vi "ziExample-Module-MDS_DAQ.vi"() -> ()   [LabVIEW 2009]
doc: "This examples allows to control a Zurich Instruments device via a LabOne Labview API. \nThis vi enables the multi-device synchronisation of two ZI instruments of the same family.\n\n© Zurich Instruments AG, www.zhinst.com"
uses:
  <instrlib>/Zurich Instruments LabOne/Public/Modules/ziTypeModEnum.ctl
  <instrlib>/Zurich Instruments LabOne/Public/Modules/ziModSetValueDouble.vi
  <instrlib>/Zurich Instruments LabOne/Public/Modules/ziModSetValueDoubleArray.vi
  <instrlib>/Zurich Instruments LabOne/Public/Modules/ziModSetValueBinary.vi
  <instrlib>/Zurich Instruments LabOne/Public/Modules/ziModGetDoubleData.vi
  <instrlib>/Zurich Instruments LabOne/Public/Utility/ziTicksToS_vector.vi
  <instrlib>/Zurich Instruments LabOne/Zurich Instruments LabOne.lvlib
panel:
  in  "subscribe":string[](array[string])=["demods/0/sample.R", "demods/0/sample.AuxIn1"] caption="Subscribe Paths"
  out "DoubleSample":T1
  in  "stop":bool
  out "XY Graph":cluster{"Timestamp(s)":dbl[], "Value":dbl[]}[](graph)
  in  "noofpoints":i32=10 caption="Number of Points"
  in  "duration":dbl=1.0 caption="Duration (s)"
  out "Error Out":errorcluster
  in  "Slaves":string[](array[string])=["dev"]
  out "Status":dbl
  out "Message":string
  in  "Master":string="dev"
  # "ziExample-Module-MDS_DAQ.vi\nRequirements: 2x(MFLI or UHF or HDAWG )\nsee block diagram for VI description"
  # "Tested Devices:\n\n- MFLI\n- UHF"
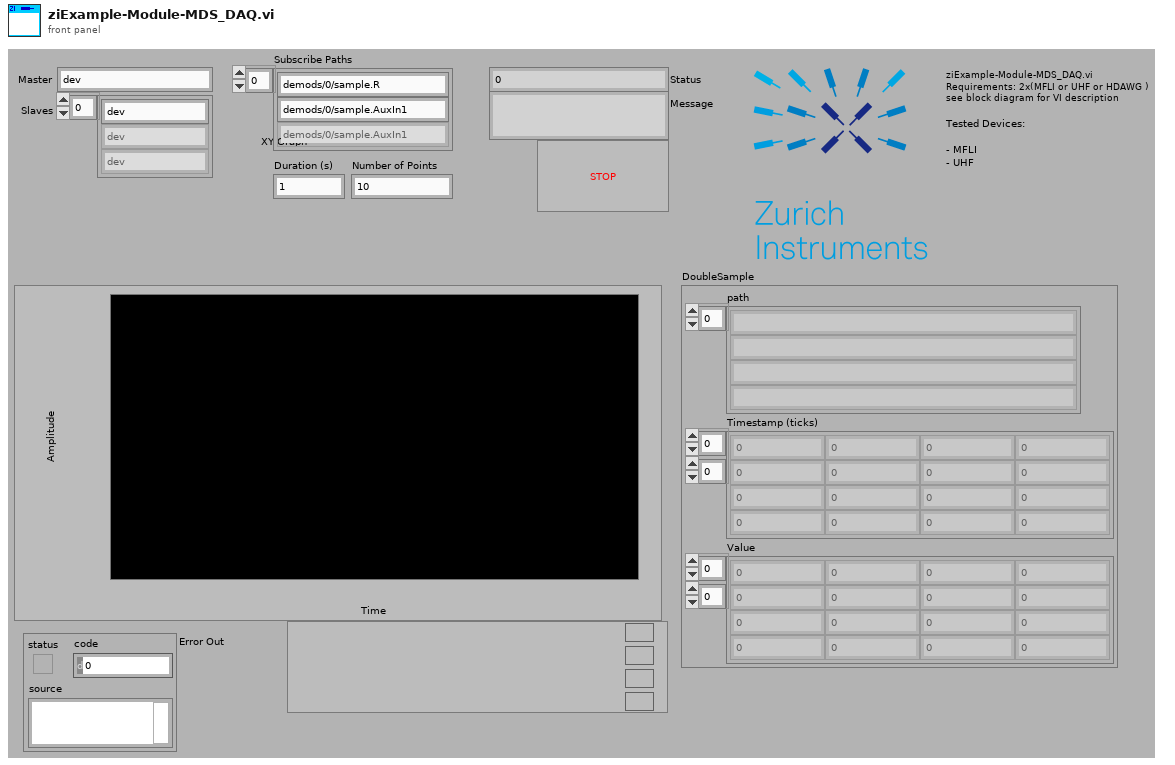
[diagram p1: front panel]
types:
  T1 = cluster{"path":string[], "Timestamp (ticks)":u64[][], "Value":dbl[][]}
  T2 = typedef "Zurich Instruments LabOne.lvlib/ziTypeModEnum.ctl" = u16
  T3 = typedef "Zurich Instruments LabOne.lvlib/ziTypeHandle.ctl" = cluster{"handleValid":bool, "Conn":u64, "Path Prefix":string, "Handle":u64, "Connected":bool, "Clockbase(s)":dbl}
  T4 = typedef "Zurich Instruments LabOne.lvlib/ziTypeModHandle.ctl" = cluster{"handleValid":bool, "Conn":u64, "ModHandle":u64, "moduleID":string, "Path Prefix":string}
  T5 = typedef "Zurich Instruments LabOne.lvlib/ziTypeModResults.ctl" = cluster{"PathArray":string[], "ValueType":T6, "NoOfResults":u64, "ziGenericHeader":T7[]}
  T6 = typedef "Zurich Instruments LabOne.lvlib/ziTypePollType.ctl" = enum16{"NONE", "DOUBLE_DATA", "INTEGER_DATA", "DEMOD_SAMPLE", "SCOPE_WAVE_HF2", "AUXIN_SAMPLE", "DIO_SAMPLE", "BYTE_ARRAY", "PWA_WAVE", "9", "10", "11", "12", "13", "14", "15", "TREE_CHANGE_DEPRI", "17", "ERROR", "19", "20", "21", "22", "23", "24", "25", "26", "27", "28", "29", "30", "31", "DOUBLE_DATA_TS", "INTEGER_DATA_TS", "34", "SCOPE_WAVE", "SCOPE_WAVE_EX", "37", "BYTE_ARRAY_TS", "39", "40", "41", "42", "43", "44", "45", "CNT_DATA", "47", "TREE_CHANGE", "49", "50", "51", "52", "53", "54", "55", "56", "57", "58", "59", "60", "61", "62", "63", "SWEEPER_DATA", "SPECTRUM_DATA", "ADVISOR_DATA", "VECTOR_DATA", "IMP_DATA"}
  T7 = typedef "Zurich Instruments LabOne.lvlib/ziTypeModGenericHeader.ctl" = cluster{"HeaderType":enum8{"HEADER_TYPE_NONE", "HEADER_TYPE_SWTRIGGER", "HEADER_TYPE_SWEEPER"}, "SampleFormat":u8, "SystemTime":timestamp, "CreatedTimeStamp":u64, "ChangedTimeStamp":u64, "Flags":u32, "ChunkSizeBytes":u64, "Name":string, "Status":u32, "GroupIndex":u32, "Color":u32, "ActiveRow":u32, "TriggerNumber":u64, "GridRows":u32, "GridCols":u32, "GridMode":u32, "GridOperation":u32, "GridDirection":u32, "GridRepetitions":u32, "GridColDelta":dbl, "GridColOffset":dbl, "GridRowDelta":dbl, "GridRowOffset":dbl, "Bandwidth":dbl, "Center":dbl, "Nenbw":dbl}
  T8 = typedef "Zurich Instruments LabOne.lvlib/ziTypeDoubleDataTS.ctl" = cluster{"Timestamp (ticks)":u64[], "Value":dbl[]}
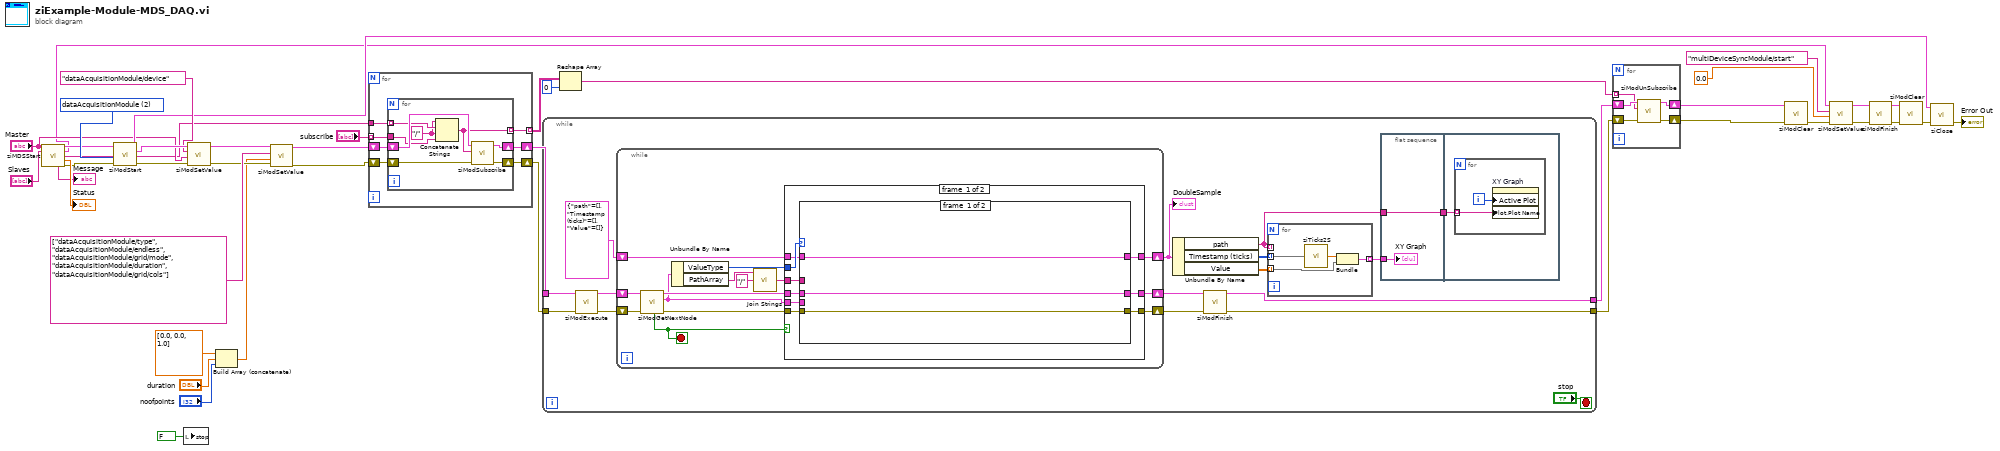
[diagram p0: block diagram]
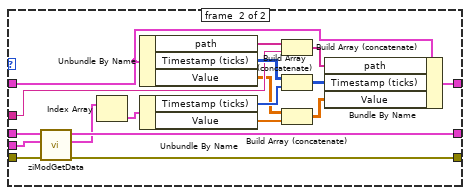
[diagram p2: hidden frame]
diagram:
  w20 = T2 2 items=["sweep", "scopeModule", "dataAcquisitionModule", "pidAdvisor", "awgModule", "impedanceModule", "multiDeviceSyncModule", "zoomFFT", "trigger", "deviceSettings", "record"] ("module Id")
  n1 = call <instrlib>:"ziMDSStart.vi"("Master"="Master", "Slaves"="Slaves") -> ("Handle Out"=w14:T3, "ModHandle Out"=w6:T4, "MDS_Devices"=w10:string[], "Status"=→"Status":dbl, "Message"=→"Message":string, "Error Out"=w13:errorcluster)  [unwired: 8 in]
  n2 = call <instrlib>:"ziModStart.vi"("Error In"=w13, "module Id"=w20, "Handle In"=w14) -> ("Error Out"=w34:errorcluster, "ModHandle Out"=w35:T4, "Handle Out"=w16:T3)  [unwired: 6 in]
  n3 = local write "stop"(FALSE ("run")) -> ()
  n4 = call-poly <instrlib>:"ziModSetValue.vi"("Error In"=w34, "Data"="Master", "Path"="dataAcquisitionModule/device", "ModHandle In"=w35) -> ("Error Out"=w29:errorcluster, "ModHandle Out"=w30:T4)  [unwired: 6 in]
  n5 = Build Array (concatenate)(dbl[] [0.0, 0.0, 1.0], "duration", "noofpoints") -> (w21:dbl[])
  n6 = call-poly <instrlib>:"ziModSetValue.vi"("Error In"=w29, "Values"=w21, "Paths"=string[] ["dataAcquisitionModule/type", "dataAcquisitionModule/endless", "dataAcquisitionModule/grid/mode", "dataAcquisitionModule/duration", "dataAcquisitionModule/grid/cols"], "ModHandle In"=w30) -> ("Error Out"=w25:errorcluster, "ModHandle Out"=w26:T4)  [unwired: 6 in]
  n7 = for {
    tunnel: "subscribe" -> [w45] mode=indexing
    shift-right: [w49] -> w28
    shift-left: w26 -> [w47]
    shift-right: [w48] -> w27
    shift-left: w25 -> [w46]
    tunnel: w10 -> [w44]
    tunnel: [w43] -> w9 mode=indexing
    n8 = for {
      tunnel: w45 -> [w51]
      tunnel: w44 -> [w53] mode=indexing
      shift-right: [w56] -> w48
      shift-left: w46 -> [w54]
      shift-right: [w57] -> w49
      shift-left: w47 -> [w55]
      tunnel: [w50] -> w43 mode=indexing
      w52 = "/" ("string")
      n9 = Concatenate Strings(w52, w53, w52, w51) -> (w50:string)
      n10 = call <instrlib>:"ziModSubscribe.vi"("Error In"=w54, "Path"=w50, "ModHandle In"=w55) -> ("Error Out"=w56:errorcluster, "ModHandle Out"=w57:T4)  [unwired: 6 in]
    }
  }
  n11 = while {
    tunnel: [w61] -> w33
    tunnel: [w71] -> w32
    tunnel: w28 -> [w70]
    tunnel: w27 -> [w69]
    stop <- "stop" stop-if-true
    n12 = call <instrlib>:"ziModExecute.vi"("Error In"=w69, "ziModHandle In"=w70) -> ("Error Out"=w67:errorcluster, "ziModHandle Out"=w68:T4)  [unwired: 6 in, 1 out]
    n13 = while {
      shift-right: [w91] -> w72
      shift-left: w68 -> [w95]
      shift-right: [w92] -> w73
      shift-left: w67 -> [w96]
      shift-right: [w84] -> w65
      shift-left: T1 {"path"=[], "Timestamp (ticks)"=[], "Value"=[]} ("DoubleSample") -> [w85]
      stop <- w90 stop-if-true
      n14 = call <instrlib>:"ziModGetNextNode.vi"("Error In"=w96, "ModHandle In"=w95) -> ("Error Out"=w93:errorcluster, "ModResults"=w89:T5, "ModHandle Out"=w94:T4, "NoData"=w90:bool)  [unwired: 6 in]
      n15 = Unbundle By Name(w89) -> ("ValueType"=w86:T6, "PathArray"=w83:string[])
      n16 = call <vilib>:"Join Strings.vi"("Separator (,)"="/", "Strings In"=w83) -> ("String"=w87:string)  [unwired: 1 in]
      n17 = case shown="False" w90 {
        tunnel: w89 -> [w105 _]
        tunnel: w94 -> [w104 w129]
        tunnel: w93 -> [w103 w128]
        tunnel: [w102 w128] -> w92
        tunnel: [w101 w129] -> w91
        tunnel: w87 -> [w97 _]
        tunnel: w86 -> [w100 _]
        tunnel: w85 -> [w99 w127]
        tunnel: [w98 w127] -> w84
        frame #0 {
          n18 = case shown="\"DOUBLE_DATA_TS\"" w100 {
            tunnel: w104 -> [w108 w123]
            tunnel: w105 -> [_ w122]
            tunnel: w103 -> [w107 w124]
            tunnel: [w107 w125] -> w102
            tunnel: [w108 w126] -> w101
            tunnel: w99 -> [w106 w112]
            tunnel: [w106 w113] -> w98
            tunnel: w97 -> [_ w115]
            frame #0 {
            }
            frame #1 {
              n19 = call-poly <instrlib>:"ziModGetData.vi"("Error In"=w124, "ModResults"=w122, "ModHandle In"=w123) -> ("Error Out"=w125:errorcluster, "DoubleSample"=w121:T8[], "ModHandle Out"=w126:T4)  [unwired: 4 in, 2 out]
              n20 = Index Array(array=w121) -> (element=w120:T8)  [unwired: 1 in]
              n21 = Unbundle By Name(w112) -> ("path"=w116:string[], "Timestamp (ticks)"=w119:u64[][], "Value"=w111:dbl[][])
              n22 = Unbundle By Name(w120) -> ("Timestamp (ticks)"=w118:u64[], "Value"=w110:dbl[])
              n23 = Build Array (concatenate)(w116, w115) -> (w114:string[])
              n24 = Build Array (concatenate)(w119, w118) -> (w117:u64[][])
              n25 = Build Array (concatenate)(w111, w110) -> (w109:dbl[][])
              n26 = Bundle By Name(cluster=w112, "path"=w114, "Timestamp (ticks)"=w117, "Value"=w109) -> (w113:T1)
            }
          }
        }
        frame #1 {
        }
      }
    }
    "DoubleSample" <- w65
    n27 = Unbundle By Name(w65) -> ("path"=w59:string[], "Timestamp (ticks)"=w64:u64[][], "Value"=w63:dbl[][])
    n28 = call <instrlib>:"ziModFinish.vi"("Error In"=w73, "ziModHandle In"=w72) -> ("Error Out"=w61:errorcluster, "ziModHandle Out"=w71:T4)  [unwired: 7 in]
    n29 = for {
      tunnel: w64 -> [w80] mode=indexing
      tunnel: w63 -> [w82] mode=indexing
      tunnel: [w81] -> w62 mode=indexing
      tunnel: w59 -> [_] mode=indexing
      n30 = call-poly <instrlib>:"ziTicks2S.vi"("Timestamp (ticks)"=w80) -> ("Timestamp(s)"=w79:dbl[])  [unwired: 2 in, 2 out]
      n31 = Bundle("Timestamp(s)"=w79, "Value"=w82) -> (w81:cluster{"Timestamp(s)":dbl[], "Value":dbl[]})  [unwired: 1 in]
    }
    n32 = flat-sequence {
      tunnel: w62 -> [w75]
      tunnel: [w74] -> w60
      tunnel: w59 -> [w74]
      tunnel: w60 -> [w76]
      frame #0 {
        "XY Graph" <- w75
      }
      frame #1 {
        n33 = for {
          tunnel: w76 -> [w78] mode=indexing
          i -> [w77]
          n34 = property on="XY Graph" class="XYGraph (strict)"("Active Plot"=w77, "Plot.Plot Name"=w78) -> ()  [unwired: 2 in, 2 out]
        }
      }
    }
  }
  n35 = Reshape Array(w9, 0 ("dimension size")) -> (w8:string[])
  n36 = for {
    tunnel: w8 -> [w130] mode=indexing
    shift-right: [w133] -> w37
    shift-left: w32 -> [w131]
    shift-right: [w134] -> w38
    shift-left: w33 -> [w132]
    n37 = call <instrlib>:"ziModUnSubscribe.vi"("Error In"=w132, "Path (\"/\")"=w130, "ModHandle In"=w131) -> ("Error Out"=w134:errorcluster, "ModHandle Out"=w133:T4)  [unwired: 7 in]
  }
  n38 = call <instrlib>:"ziModClear.vi"("Error In"=w38, "ziModHandle In"=w37) -> ("Error Out"=w3:errorcluster)  [unwired: 7 in, 1 out]
  n39 = call-poly <instrlib>:"ziModSetValue.vi"("Error In"=w3, "Value"=0.0, "Path"="multiDeviceSyncModule/start", "ModHandle In"=w6) -> ("Error Out"=w2:errorcluster, "ModHandle Out"=w5:T4)  [unwired: 6 in]
  n40 = call <instrlib>:"ziModFinish.vi"("Error In"=w2, "ziModHandle In"=w5) -> ("Error Out"=w42:errorcluster, "ziModHandle Out"=w41:T4)  [unwired: 7 in]
  n41 = call <instrlib>:"ziModClear.vi"("Error In"=w42, "ziModHandle In"=w41) -> ("Error Out"=w12:errorcluster)  [unwired: 7 in, 1 out]
  n42 = call <instrlib>:"ziClose.vi"("Error In"=w12, "Handle In"=w16) -> ("Error Out"=→"Error Out":errorcluster)  [unwired: 2 in, 1 out]
